vi "getPos.vi"(1 "axisIdx":i32, 2 "System no.":i32=1 min=1 max=4 step=1) -> (0 "stagePos":dbl)   [LabVIEW 2015]
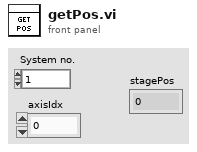
[diagram p1: front panel]
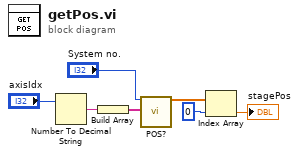
[diagram p0: block diagram]
diagram:
  n1 = Number To Decimal String(number="axisIdx") -> (decimal integer string=w6:string)  [unwired: 1 in]
  n2 = Build Array(w6) -> (w4:string[])
  n3 = call "POS?.vi"("System no."="System no.", "Axes to query"=w4) -> ("Position"=w2:dbl[])  [unwired: 16 in, 1 out]
  n4 = Index Array(array=w2, index=0) -> (element=→"stagePos":dbl)
